vi "Read Results.lvclass.vi"(8 "error in (no error)":errorcluster, 11 "Send Results Object in":refnum<class "Send Results Object.lvclass">) -> (0 "error out":errorcluster, 2 "Results.lvclass":refnum<class "Results.lvclass">, 3 "Send Results Object out":refnum<class "Send Results Object.lvclass">)   [LabVIEW 2016, in "Controller Actor.lvlib" / "Send Results Object.lvclass"]
uses:
  <userlib>/Common Components/Controller/Messages/Send Results Object/Send Results Object.lvclass
  <userlib>/Common Components/Results/Results.lvclass
  <userlib>/Common Components/Controller/Messages/Send Results Object/Send Results Object.lvclass/Send Results Object.ctl
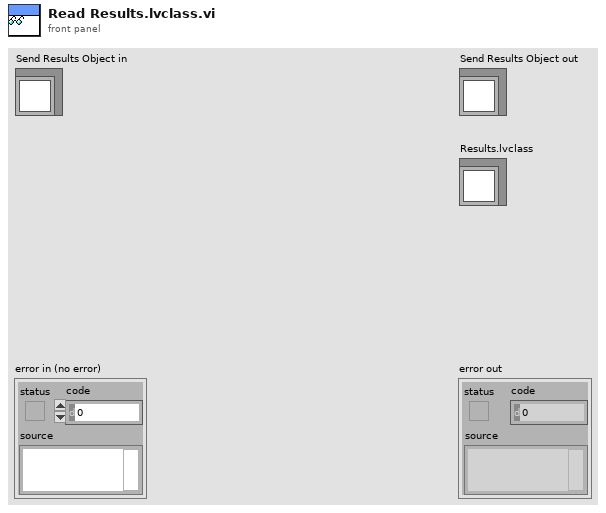
[diagram p1: front panel]
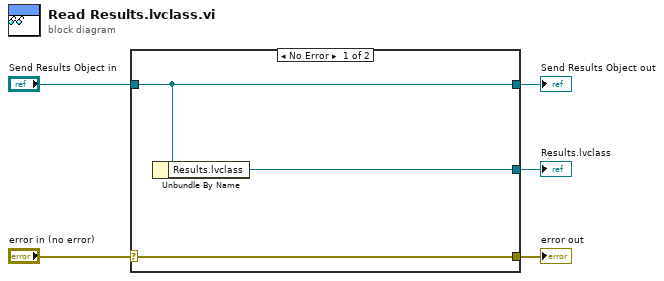
[diagram p0: block diagram]
diagram:
  n1 = case shown="No Error" "error in (no error)" {
    selector: "error in (no error)" -> [w8 w9]
    tunnel: [w8 w9] -> w4
    tunnel: [w7 w10] -> w2
    tunnel: "Send Results Object in" -> [w7 w10]
    tunnel: [w6 _] -> w1
    frame No Error {
      n2 = Unbundle By Name(w7) -> ("Results.lvclass"=w6:refnum<class "Results.lvclass">)
    }
    frame Error {
    }
  }
  "error out" <- w4
  "Send Results Object out" <- w2
  "Results.lvclass" <- w1
